vi "stats.vi"(8 "error in (no error)":errorcluster, 11 "BMC in":refnum<class "BMC.lvclass">) -> (0 "error out":errorcluster, 2 "actuator array":dbl[](array[numeric]), 3 "BMC out":refnum<class "BMC.lvclass">)   [LabVIEW 2012, in "BMC.lvclass"]
uses:
  BMC.lvclass
  BMC.lvclass/BMC.ctl
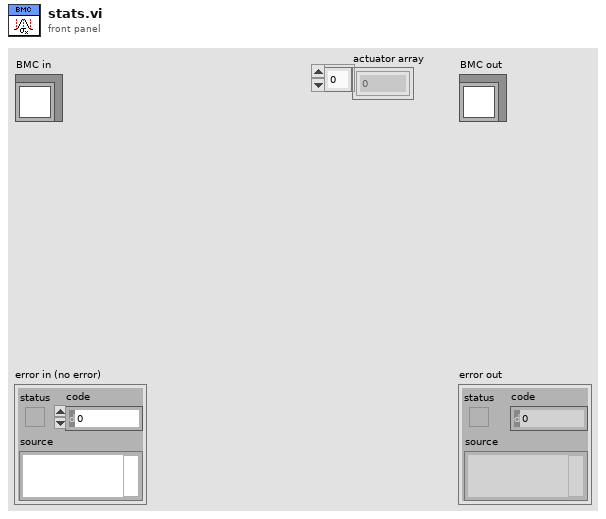
[diagram p1: front panel]
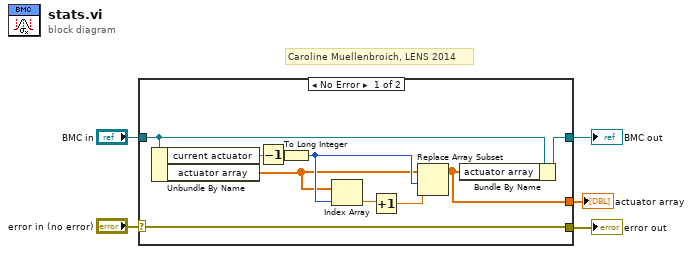
[diagram p0: block diagram]
diagram:
  # "Caroline Muellenbroich, LENS 2014"
  n1 = case shown="No Error" "error in (no error)" {
    selector: "error in (no error)" -> [w15 w17]
    tunnel: [w15 w17] -> w4
    tunnel: [w9 w16] -> w2
    tunnel: "BMC in" -> [w10 w16]
    tunnel: [w8 _] -> w1
    frame No Error {
      n2 = Unbundle By Name(w10) -> ("current actuator"=w7:dbl, "actuator array"=w11:dbl[])
      n3 = Decrement(x=w7) -> (x-1=w6:dbl)
      n4 = To Long Integer(number=w6) -> (32bit integer=w12:i32)
      n5 = Index Array(array=w11, index=w12) -> (element=w14:dbl)
      n6 = Increment(x=w14) -> (x+1=w13:dbl)
      n7 = Replace Array Subset(array=w11, new element=w13, index=w12) -> (w8:dbl[])
      n8 = Bundle By Name(cluster=w10, "actuator array"=w8) -> (w9:refnum<class "BMC.lvclass">)
    }
    frame Error {
    }
  }
  "error out" <- w4
  "BMC out" <- w2
  "actuator array" <- w1
